vi "Read driveMode.vi"(8 "error in (no error)":errorcluster, 11 "MotorController in":refnum<class "MotorController.lvclass">) -> (0 "error out":errorcluster, 2 "driveMode":enum16{"velocityMode", "torqueMode", ""}(ring), 3 "MotorController out":refnum<class "MotorController.lvclass">)   [LabVIEW 2017, in "MotorController.lvclass"]
uses:
  MotorController.lvclass
  MotorController.lvclass/MotorController.ctl
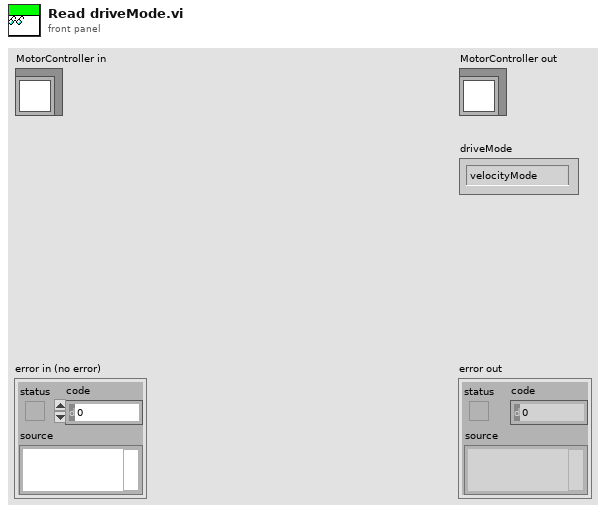
[diagram p1: front panel]
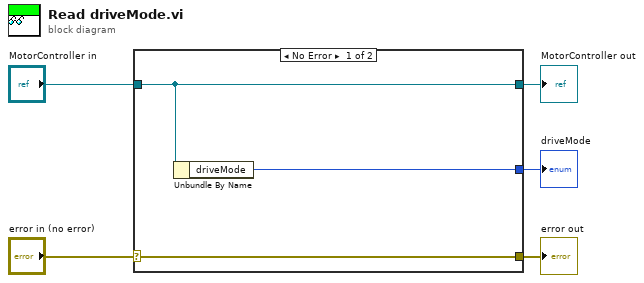
[diagram p0: block diagram]
diagram:
  n1 = case shown="No Error" "error in (no error)" {
    selector: "error in (no error)" -> [w8 w9]
    tunnel: [w8 w9] -> w4
    tunnel: [w7 w10] -> w2
    tunnel: "MotorController in" -> [w7 w10]
    tunnel: [w6 _] -> w1
    frame No Error {
      n2 = Unbundle By Name(w7) -> ("driveMode"=w6:enum16{"velocityMode", "torqueMode", ""})
    }
    frame Error {
    }
  }
  "error out" <- w4
  "MotorController out" <- w2
  "driveMode" <- w1
